vi "set_setpoint.vi"(8 "error in (no error)":errorcluster, 10 "setpoint":dbl, 11 "heat_board_control in":refnum<class "heat_board_control.lvclass">) -> (0 "error out":errorcluster, 3 "heat_board_control out":refnum<class "heat_board_control.lvclass">)   [LabVIEW 2015, in "heat_board_control.lvclass"]
uses:
  heat_board_control.lvclass
  heat_board_control.lvclass/heat_board_control.ctl
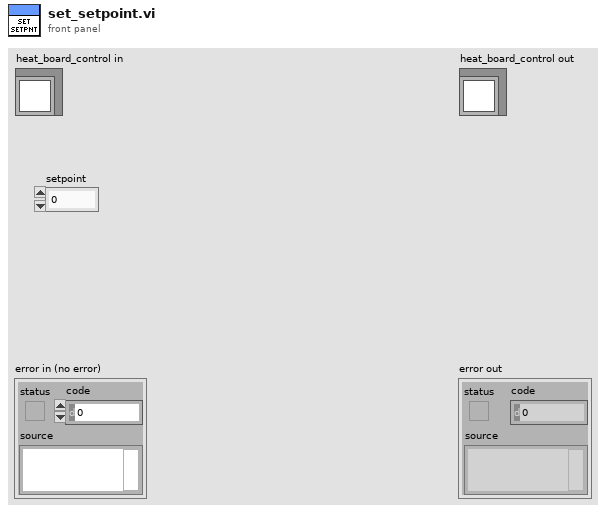
[diagram p1: front panel]
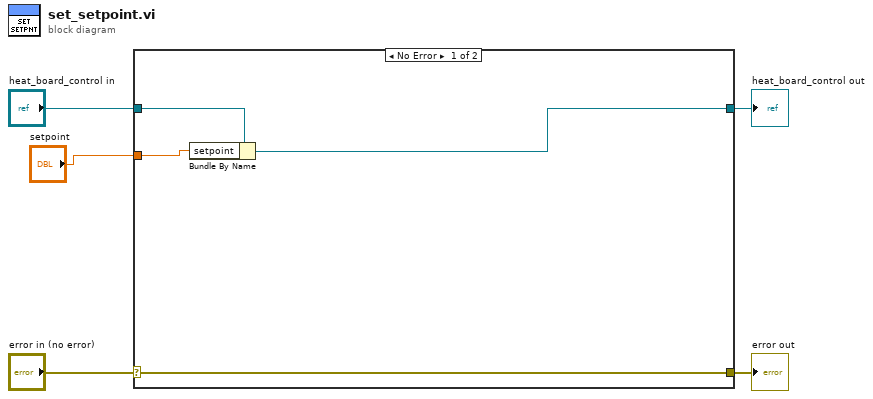
[diagram p0: block diagram]
diagram:
  n1 = case shown="No Error" "error in (no error)" {
    selector: "error in (no error)" -> [w6 w11]
    tunnel: [w6 w11] -> w4
    tunnel: [w7 w10] -> w2
    tunnel: "heat_board_control in" -> [w9 w10]
    tunnel: "setpoint" -> [w8 _]
    frame No Error {
      n2 = Bundle By Name(cluster=w9, "setpoint"=w8) -> (w7:refnum<class "heat_board_control.lvclass">)
    }
    frame Error {
    }
  }
  "error out" <- w4
  "heat_board_control out" <- w2
